vi "Create one pair.vi"(0 "Color":u32, 5 "Number":i32, 7 "XL":dbl, 9 "XR":dbl, 11 "Y":dbl) -> (4 "Cursors":T1(array[cluster]), 6 "Names":string[](array[string]), 8 "Xs":dbl[](array[numeric]))   [LabVIEW 2014, in "Graph with cursors XControl.xctl"]
uses:
  Graph with cursors XControl.xctl
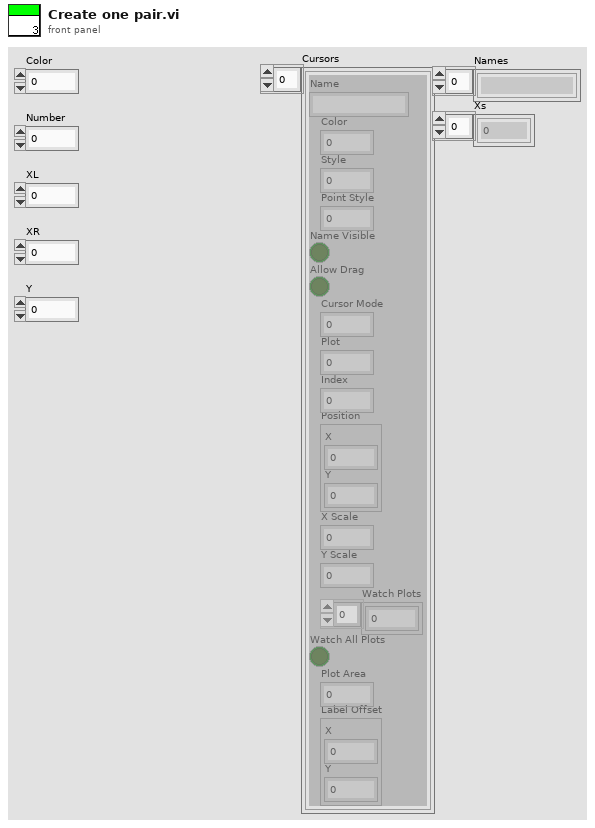
[diagram p1: front panel]
types:
  T1 = cluster{"Name":string, "Color":u32, "Style":u8, "Point Style":u8, "Name Visible":bool, "Allow Drag":bool, "Cursor Mode":u32, "Plot":i32, "Index":i32, "Position":cluster{"X":dbl, "Y":dbl}, "X Scale":u32, "Y Scale":u32, "Watch Plots":i32[], "Watch All Plots":bool, "Plot Area":i32, "Label Offset":cluster{"X":dbl, "Y":dbl}}[]
  T2 = cluster{"Name":string, "Color":u32, "Style":u8, "Point Style":u8, "Name Visible":bool, "Allow Drag":bool, "Cursor Mode":u32, "Plot":i32, "Index":i32, "Position":cluster{"X":dbl, "Y":dbl}, "X Scale":u32, "Y Scale":u32, "Watch Plots":i32[], "Watch All Plots":bool, "Plot Area":i32, "Label Offset":cluster{"X":dbl, "Y":dbl}}
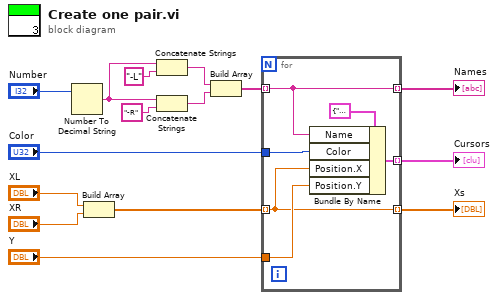
[diagram p0: block diagram]
diagram:
  n1 = Number To Decimal String(number="Number") -> (decimal integer string=w12:string)  [unwired: 1 in]
  n2 = Build Array("XL", "XR") -> (w7:dbl[])
  n3 = Concatenate Strings(w12, "-L" ("string")) -> (w10:string)
  n4 = Concatenate Strings(w12, "-R" ("string")) -> (w11:string)
  n5 = Build Array(w10, w11) -> (w6:string[])
  n6 = for {
    tunnel: w7 -> [w17] mode=indexing
    tunnel: w6 -> [w16] mode=indexing
    tunnel: "Y" -> [w19]
    tunnel: "Color" -> [w20]
    tunnel: [w18] -> w3 mode=indexing
    tunnel: [w17] -> w1 mode=indexing
    tunnel: [w16] -> w2 mode=indexing
    n7 = Bundle By Name(cluster=T2 {"Name"="", "Color"=16711680, "Style"=2, "Point Style"=0, "Name Visible"=TRUE, "Allow Drag"=TRUE, "Cursor Mode"=0, "Plot"=0, "Index"=0, "Position"={"X"=0.0, "Y"=0.0}, "X Scale"=0, "Y Scale"=0, "Watch Plots"=[], "Watch All Plots"=FALSE, "Plot Area"=0, "Label Offset"={"X"=0.0, "Y"=0.0}} ("element"), "Name"=w16, "Color"=w20, "Position.X"=w17, "Position.Y"=w19) -> (w18:T2)
  }
  "Cursors" <- w3
  "Names" <- w2
  "Xs" <- w1
